vi "ClienteSimples.vi"(2 "remote port":u16=4848, 5 "error in (no error)":errorcluster) -> (16 "value":T1[](array[typedef]), 19 "error out":errorcluster)   [LabVIEW 2012, in "SimusinClient.lvlib"]
uses:
  SimusinClient.lvlib
  Typedefs/Tipo_PacoteModuloCRIO.ctl
  Typedefs/Tipo_moduloCRIO.ctl
  <vilib>/NI/STM/TCP/Read Meta Data (TCP Ref).vi
  <vilib>/NI/STM/TCP/Write Message (TCP).vi
  <vilib>/NI/STM/TCP/Read Message (TCP).vi
  <vilib>/NI/STM/TCP/Read Meta Data (TCP Clst).vi
  <vilib>/NI/STM/NI STM.lvlib
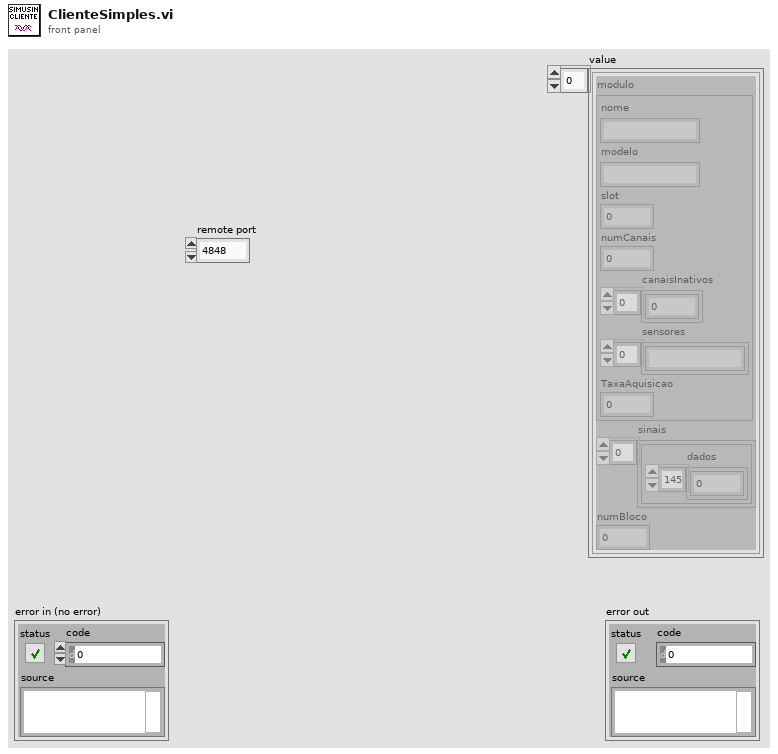
[diagram p1: front panel]
types:
  T1 = typedef "Tipo_PacoteModuloCRIO.ctl" = cluster{"modulo":T2, "sinais":cluster{"dados":sgl[]}[], "numBloco":i32}
  T2 = typedef "Tipo_moduloCRIO.ctl" = cluster{"nome":string, "modelo":string, "slot":i32, "numCanais":i32, "canaisInativos":i32[], "sensores":string[], "TaxaAquisicao":dbl}
  T3 = typedef "NI STM.lvlib/TCP Connection Info.ctl" = cluster{"connection ID":refnum<k5>, "meta data":T4[]}
  T4 = typedef "NI STM.lvlib/MetaDataElement.ctl" = string
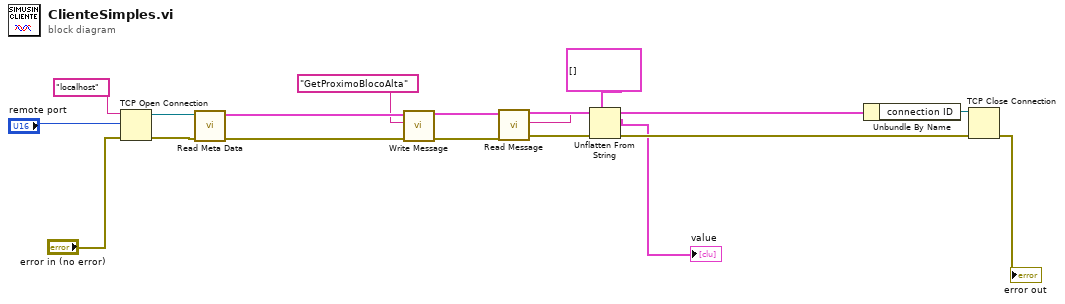
[diagram p0: block diagram]
diagram:
  n1 = TCP Open Connection(address="localhost" ("Target IP Address"), remote port or service name="remote port", error in (no error)="error in (no error)") -> (connection ID=w16:refnum<k5>, error out=w15:errorcluster)  [unwired: 2 in]
  n2 = call-poly <vilib>:"Read Meta Data.vi"("error in"=w15, "connection ID"=w16) -> ("error out"=w13:errorcluster, "connection info out"=w14:T3)  [unwired: 7 in, 1 out]
  n3 = call-poly <vilib>:"Write Message.vi"("error in"=w13, "name"="GetProximoBlocoAlta", "connection info in"=w14) -> ("error out"=w7:errorcluster, "connection info out"=w8:T3)  [unwired: 7 in]
  n4 = call-poly <vilib>:"Read Message.vi"("error in"=w7, "connection info in"=w8) -> ("error out"=w5:errorcluster, "data string"=w6:string, "connection info out"=w11:T3)  [unwired: 4 in, 3 out]
  n5 = Unflatten From String(type=T1[] [], binary string=w6, error in (no error)=w5) -> (value=→"value":T1[], error out=w12:errorcluster)  [unwired: 2 in, 1 out]
  n6 = Unbundle By Name(w11) -> ("connection ID"=w10:refnum<k5>)
  n7 = TCP Close Connection(connection ID=w10, error in (no error)=w12) -> (error out=→"error out":errorcluster)  [unwired: 1 in, 1 out]
